vi "2_Control LED using Push Button.vi"() -> ()   [LabVIEW 2018]
panel:
  out "Round LED":bool
  in  "Push Button":bool
  # "Develop HMI to control LED using Push Button"
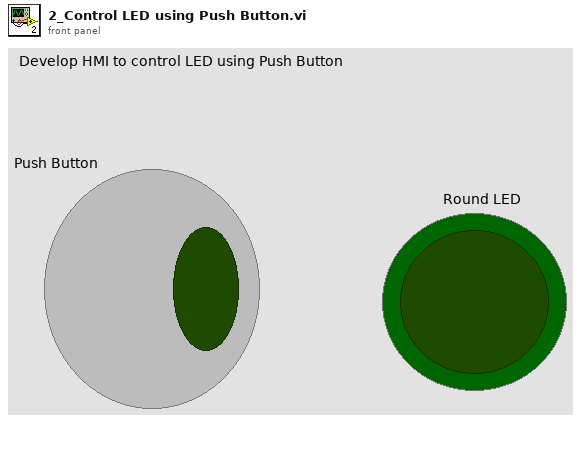
[diagram p1: front panel]
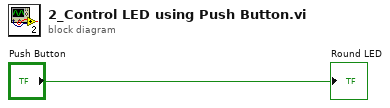
[diagram p0: block diagram]
diagram:
  "Round LED" <- "Push Button"
